vi "AOL Z Cal-Base string.vi"(4 "Norm coord for cal process":dbl=-0.8, 5 "Number of FOVs":i32=3, 6 "Initial motor Z":sgl=172.0, 7 "Index of current FOV":i32=2, 8 "Index of current Cal point":i32=15, 9 "Number of Cal points (per FOV)":i32=21, 11 "FOV (string)":string="235") -> (2 "Progress %":u8=255)   [LabVIEW 2020]
uses:
  Globals/gl_Calibration globals.vi
panel:
  out "Base String":string
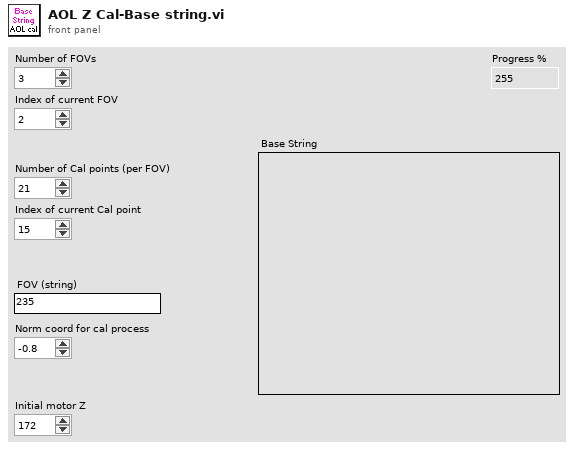
[diagram p1: front panel]
types:
  T1 = typedef "Cal mode.ctl" = enum16{"Automatic", "Interactive"}
  T2 = typedef "AOL Z cal process refs.ctl" = cluster{"This VI":refnum<vi>, "Abort (ind)":refnum<vi>, "Next (ind)":refnum<vi>, "Cancel":refnum<vi>, "Next":refnum<vi>, "Message":refnum<vi>, "Progress":refnum<vi>}
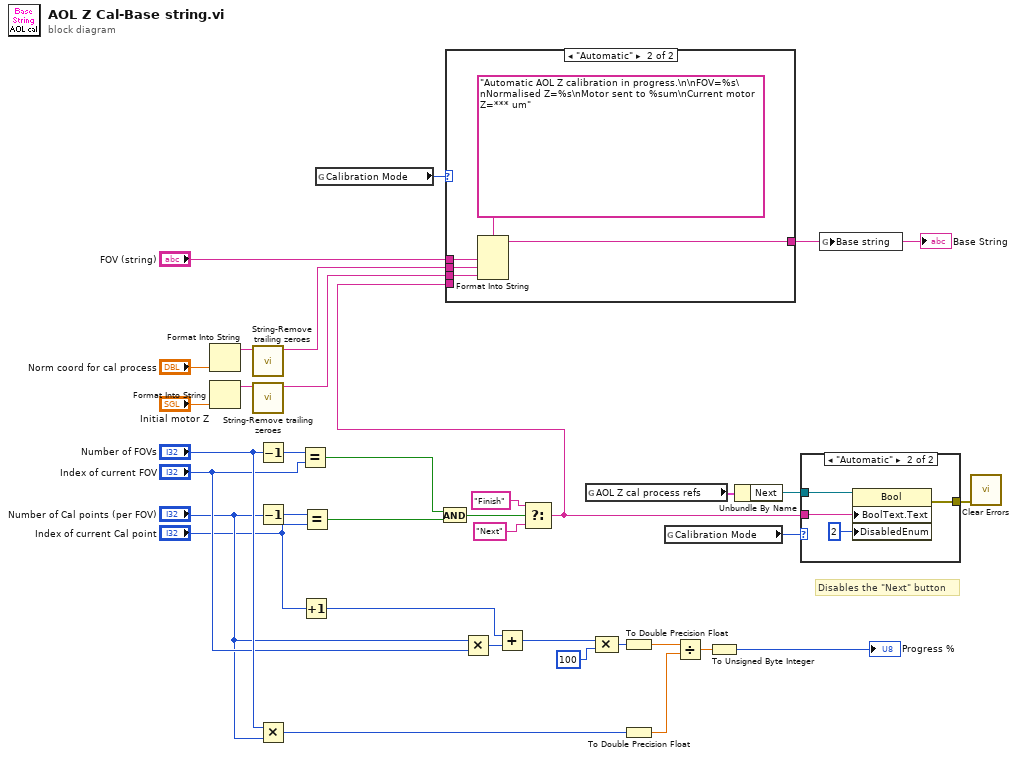
[diagram p0: block diagram]
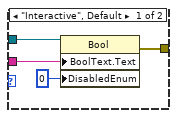
[diagram p2: hidden frame]
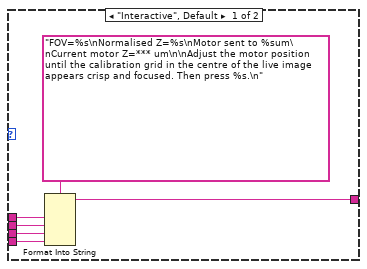
[diagram p3: hidden frame]
diagram:
  # "Disables the \"Next\" button"
  n1 = Format Into String("Norm coord for cal process") -> (resulting string=w29:string)  [unwired: 3 in, 1 out]
  n2 = Format Into String("Initial motor Z") -> (resulting string=w34:string)  [unwired: 3 in, 1 out]
  n3 = call <userlib>:"String-Remove trailing zeroes.vi"("String in"=w29) -> ("String out"=w4:string)  [unwired: 10 in]
  n4 = call <userlib>:"String-Remove trailing zeroes.vi"("String in"=w34) -> ("String out"=w3:string)  [unwired: 10 in]
  n5 = Decrement(x="Number of FOVs") -> (x-1=w24:i32)
  n6 = Decrement(x="Number of Cal points (per FOV)") -> (x-1=w23:i32)
  n7 = Multiply(x="Number of FOVs", y="Number of Cal points (per FOV)") -> (x*y=w17:i32)
  n8 = Equal?(x=w24, y="Index of current FOV") -> (x = y?=w22:bool)
  n9 = Increment(x="Index of current Cal point") -> (x+1=w6:i32)
  n10 = Equal?(x=w23, y="Index of current Cal point") -> (x = y?=w12:bool)
  n11 = global read "gl_Calibration globals.vi" "Calibration Mode"() -> (w26:T1)
  n12 = And(x=w22, y=w12) -> (x .and. y?=w31:bool)
  n13 = Multiply(x="Number of Cal points (per FOV)", y="Index of current FOV") -> (x*y=w8:i32)
  n14 = Add(x=w6, y=w8) -> (x+y=w9:i32)
  n15 = Select(t="Finish" ("Boolean Text.Text"), s=w31, f="Next" ("Boolean Text.Text")) -> (s? t:f=w2:string)
  n16 = case shown="\"Automatic\"" w26 {
    tunnel: "FOV (string)" -> [w40 w46]
    tunnel: w4 -> [w39 w44]
    tunnel: w3 -> [w38 w43]
    tunnel: w2 -> [w37 _]
    tunnel: [w36 w42] -> w1
    frame "Interactive", Default {
      n17 = Format Into String(format string="FOV=%s\nNormalised Z=%s\nMotor sent to %sum\nCurrent motor Z=*** um\n\nAdjust the motor position until the calibration grid in the centre of the live image appears crisp and focused. Then press %s.\n", w40, w39, w38, w37) -> (resulting string=w36:string)  [unwired: 2 in, 1 out]
    }
    frame "Automatic" {
      n18 = Format Into String(format string="Automatic AOL Z calibration in progress.\n\nFOV=%s\nNormalised Z=%s\nMotor sent to %sum\nCurrent motor Z=*** um", w46, w44, w43) -> (resulting string=w42:string)  [unwired: 2 in, 1 out]
    }
  }
  "Base String" <- w1
  n19 = global read "gl_Calibration globals.vi" "AOL Z cal process refs"() -> (w28:T2)
  n20 = Compound Arithmetic op=MULTIPLY(w9, 100 ("value")) -> (w19:i32)
  n21 = To Double Precision Float(number=w19) -> (double precision float=w18:dbl)
  n22 = To Double Precision Float(number=w17) -> (double precision float=w16:dbl)
  n23 = global read "gl_Calibration globals.vi" "Calibration Mode"() -> (w25:T1)
  n24 = Divide(x=w18, y=w16) -> (x/y=w15:dbl)
  n25 = To Unsigned Byte Integer(number=w15) -> (unsigned 8bit integer=→"Progress %":u8)
  n26 = Unbundle By Name(w28) -> ("Next"=w27:refnum<vi>)
  n27 = case shown="\"Automatic\"" w25 {
    tunnel: w27 -> [w50 w54]
    tunnel: w2 -> [w49 w53]
    tunnel: [w47 w51] -> w14
    frame "Interactive", Default {
      n28 = property on="Property Node" class="Bool"(reference=w50, "BoolText.Text"=w49, "DisabledEnum"=0) -> (error out=w47:errorcluster)  [unwired: 1 in, 1 out]
    }
    frame "Automatic" {
      n29 = property on="Property Node" class="Bool"(reference=w54, "BoolText.Text"=w53, "DisabledEnum"=2) -> (error out=w51:errorcluster)  [unwired: 1 in, 1 out]
    }
  }
  n30 = global write "gl_Calibration globals.vi" "Base string"(w1) -> ()
  n31 = call <vilib>:"Clear Errors.vi"("error in (no error)"=w14) -> ()  [unwired: 5 in, 2 out]
